vi "Load SVG From File (Core).vi"(8 "error in (no error)":errorcluster, 10 "Scale (1)":dbl=1.0, 11 "Path In":string) -> (0 "error out":errorcluster, 2 "Extended Image":T1, 3 "Path Out":string)   [LabVIEW 2020, in "G-Image.lvlib"]
doc: "Load an image file from disk."
uses:
  G-Image.lvlib
  Private/Extended Image.ctl
  <vilib>/picture/picture.llb/imagedata.ctl
  <vilib>/Utility/error.llb/Error Cluster From Error Code.vi
  lib/g_image_32.dll
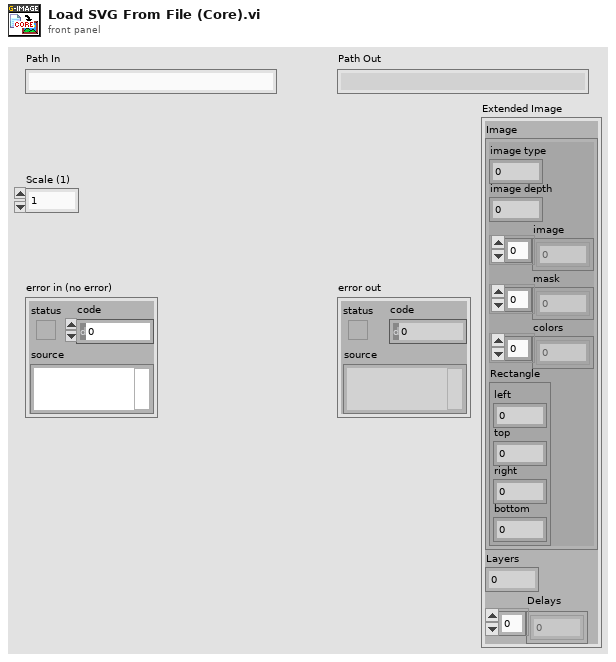
[diagram p1: front panel]
types:
  T1 = typedef "G-Image.lvlib/Extended Image.ctl" = cluster{"Image":T2, "Layers":i32, "Delays":i32[]}
  T2 = typedef "imagedata.ctl" = cluster{"image type":i32, "image depth":i32, "image":u8[], "mask":u8[], "colors":u32[], "Rectangle":cluster{"left":i16, "top":i16, "right":i16, "bottom":i16}}
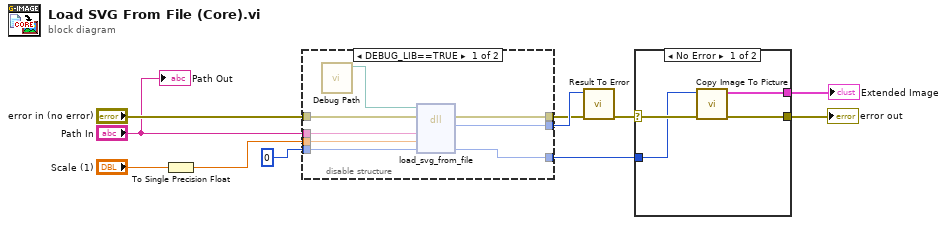
[diagram p0: block diagram]
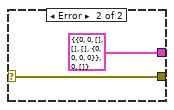
[diagram p2: hidden frame]
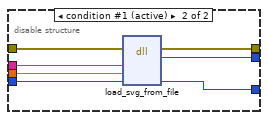
[diagram p3: hidden frame]
diagram:
  n1 = To Single Precision Float(number="Scale (1)") -> (single precision float=w1:sgl)
  n2 = disable-structure shown="DEBUG_LIB==TRUE" {
    disable-tunnel: [w18 w26] -> w8
    disable-tunnel: "error in (no error)" -> [w17 w25]
    disable-tunnel: "Path In" -> [w16 w24]
    disable-tunnel: [w15 w23] -> w9
    disable-tunnel: [w14 w21] -> w4
    disable-tunnel: i64 0 ("count") -> [w13 w22]
    disable-tunnel: w1 -> [w12 w20]
    frame condition #0 {
      n3 = call "Debug Path.vi"() -> ("Debug Path"=w19:path)  [unwired: 11 in]
      n4 = dll-call lib="?" fn="load_svg_from_file"(path in=w19, error in=w17, "file_name"=w16, "scale"=w12, "image_out"=w13) -> (error out=w18:errorcluster, "result"=w15:i32, "image_out"=w14:i64)  [unwired: 3 in, 1 out]
    }
    frame condition #1 (active) {
      n5 = dll-call lib="C:/github/dataflowg/g-image/src/LabVIEW/G-Image/lib/g_image_*.*" fn="load_svg_from_file"(error in=w25, "file_name"=w24, "scale"=w20, "image_out"=w22) -> (error out=w26:errorcluster, "result"=w23:i32, "image_out"=w21:i64)  [unwired: 4 in, 1 out]
    }
  }
  n6 = call "Result To Error.vi"("error in (no error)"=w8, "Result Code"=w9) -> ("error out"=w7:errorcluster)  [unwired: 9 in]
  n7 = case shown="No Error" w7 {
    selector: w7 -> [w30 w32]
    tunnel: [w28 w32] -> w11
    tunnel: w4 -> [w29 _]
    tunnel: [w27 T1 {"Image"={"image type"=0, "image depth"=0, "image"=[], "mask"=[], "colors"=[], "Rectangle"={"left"=0, "top"=0, "right"=0, "bottom"=0}}, "Layers"=0, "Delays"=[]} ("Image")] -> w3
    frame No Error {
      n8 = call "Copy Image To Picture.vi"("error in (no error)"=w30, "image_ptr"=w29) -> ("error out"=w28:errorcluster, "Extended Image"=w27:T1)  [unwired: 8 in]
    }
    frame Error {
    }
  }
  "error out" <- w11
  "Extended Image" <- w3
  "Path Out" <- "Path In"
